vi "IVC_OC200_init_visa.vi"(8 "error in":errorcluster, 9 "termination char\n(0xA = '\\n' = LF)":u8=10 format="%.0x", 10 "Mask":T1=16 items=["Flush Receive Buffer"=16, "Write Transmit Buffer to Device"=32, "Flush Receive Buffer (No I/O)"=64, "Flush Transmit Buffer"=128], 11 "VISA resource name":refnum<visa-resource-name>) -> (0 "error out":errorcluster, 3 "VISA resource name out":refnum<visa-resource-name>, 6 ".not. x?":bool)   [LabVIEW 2019]
uses:
  <vilib>/Instr/_visa.llb/VISA Flush IO Buffer Mask.ctl
  <vilib>/Instr/_visa.llb/VISA Configure Serial Port (Instr).vi
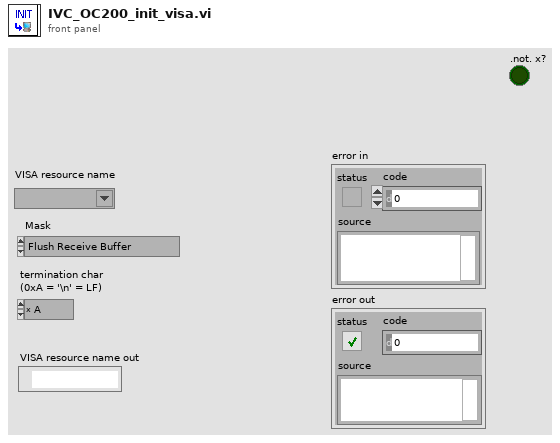
[diagram p1: front panel]
types:
  T1 = typedef "VISA Flush IO Buffer Mask.ctl" = u16
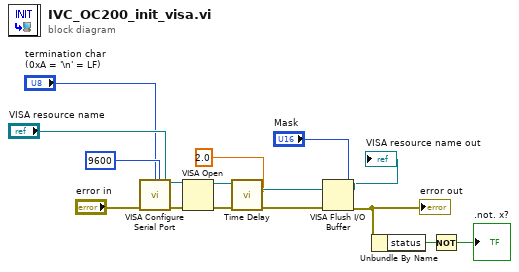
[diagram p0: block diagram]
diagram:
  n1 = call-poly "VISA Configure Serial Port"("VISA resource name"="VISA resource name", "termination char\n(0xA = '\\n' = LF)"="termination char\n(0xA = '\\n' = LF)", "baud rate (9600)"=u32 9600, "error in (no error)"="error in") -> ("VISA resource name out"=w10:refnum<visa-resource-name>, "error out"=w9:errorcluster)  [unwired: 10 in]
  n2 = VISA Open(error in (no error)=w9, VISA resource name=w10) -> (VISA resource name=w15:refnum<visa-resource-name>, error out=w5:errorcluster)  [unwired: 3 in]
  n3 = call "Time Delay"("error in (no error)"=w5, "Delay Time (s)"=2.0) -> ("error out"=w6:errorcluster)  [unwired: 9 in]
  n4 = VISA Flush I/O Buffer(VISA resource name=w15, mask (16)="Mask", error in (no error)=w6) -> (VISA resource name out=→"VISA resource name out":refnum<visa-resource-name>, error out=w2:errorcluster)
  "error out" <- w2
  n5 = Unbundle By Name(w2) -> ("status"=w3:bool)
  n6 = Not(x=w3) -> (.not. x?=→".not. x?":bool)
